vi "rasp11.vi"(7 "data type":waveform(i16)) -> (1 "element":i16)   [LabVIEW 2010]
panel:
  out "output cluster":cluster{i16[], i32[]}
  out "index":i32
  out "Waveform Graph":waveform(i16)[](graph)
  out "XY Graph":cluster{i16[], i32[]}(graph)
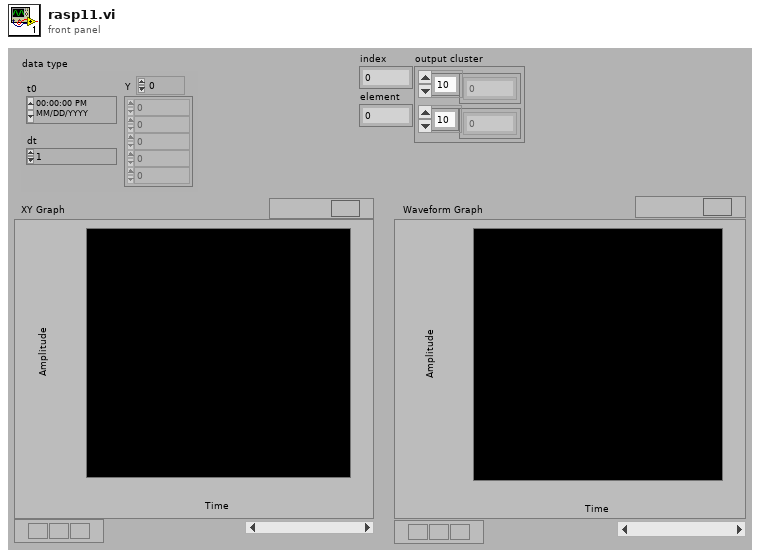
[diagram p1: front panel]
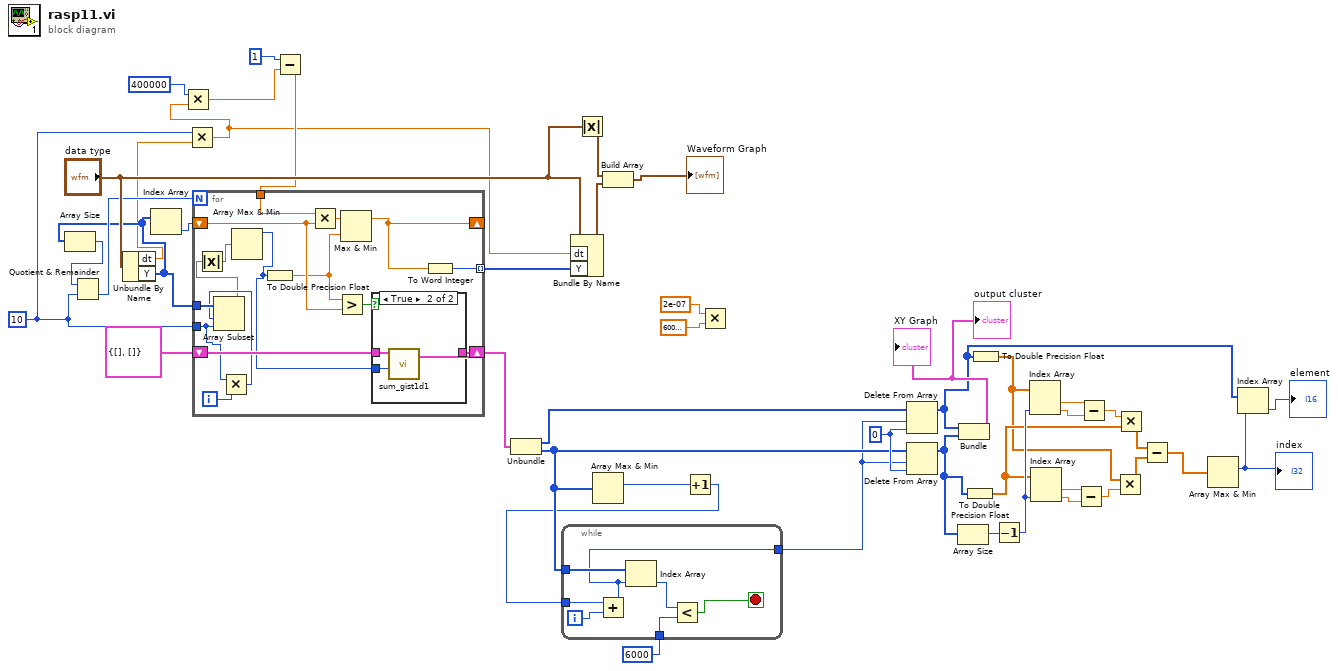
[diagram p0: block diagram]
diagram:
  w23 = 10 ("y")
  w42 = 0 ("index")
  n1 = Unbundle By Name("data type") -> ("dt"=w26:dbl, "Y"=w27:i16[])
  n2 = Array Size(array=w27) -> (size(s)=w29:i32)
  n3 = Quotient & Remainder(x=w29, y=w23) -> (floor(x/y)=w28:i32)  [unwired: 1 out]
  n4 = Index Array(array=w27) -> (element=w38:i16)  [unwired: 1 in]
  n5 = Multiply(x=w23, y=w26) -> (x*y=w1:dbl)
  n6 = Multiply(x=400000, y=w1) -> (x*y=w21:dbl)
  n7 = Subtract(x=1, y=w21) -> (x-y=w24:dbl)
  n8 = for {
    N: w28 -> [_]
    shift-right: [w54] -> _
    shift-left: w38 -> [w56]
    tunnel: [w61] -> w45 mode=indexing
    shift-right: [w59] -> w37
    shift-left: cluster{i16[], i32[]} {[], []} ("hist") -> [w60]
    tunnel: w24 -> [w53]
    tunnel: w27 -> [w52]
    tunnel: w23 -> [w50]
    i -> [w51]
    n9 = Multiply(x=w50, y=w51) -> (x*y=w49:i32)
    n10 = Array Subset(array=w52, index=w49, length=w50) -> (w48:i16[])
    n11 = Absolute Value(x=w48) -> (abs(x)=w47:i16[])
    n12 = Array Max & Min(array=w47) -> (max value=w46:i16)  [unwired: 3 out]
    n13 = To Double Precision Float(number=w46) -> (double precision float=w55:dbl)
    n14 = Multiply(x=w53, y=w56) -> (x*y=w58:dbl)
    n15 = Greater?(x=w55, y=w56) -> (0:w57:bool)
    n16 = Max & Min(x=w58, y=w55) -> (max(x,y)=w54:dbl)  [unwired: 1 out]
    n17 = case shown="True" w57 {
      tunnel: w60 -> [w62 w64]
      tunnel: w46 -> [_ w63]
      tunnel: [w62 w65] -> w59
      frame False {
      }
      frame True {
        n18 = call "sum_gist1d1.vi"("Y"=w63, "hist in"=w64) -> ("hist"=w65:cluster{i16[], i32[]})  [unwired: 3 in]
      }
    }
    n19 = To Word Integer(number=w54) -> (16bit integer=w61:i16)
  }
  n20 = Unbundle(w37) -> (w43:i16[], w36:i32[])
  n21 = Bundle By Name(cluster="data type", "dt"=w1, "Y"=w45) -> (w41:waveform(i16))
  n22 = Absolute Value(x="data type") -> (abs(x)=w40:waveform(i16))
  n23 = Array Max & Min(array=w36) -> (max index (indices)=w35:i32)  [unwired: 3 out]
  n24 = Build Array(w40, w41) -> (→"Waveform Graph":waveform(i16)[])
  n25 = Increment(x=w35) -> (x+1=w34:i32)
  n26 = while {
    tunnel: w36 -> [w72]
    tunnel: [w66] -> w33
    tunnel: 6000 ("y") -> [w70]
    tunnel: w34 -> [w67]
    i -> [w68]
    stop <- w69 stop-if-true
    n27 = Add(x=w67, y=w68) -> (x+y=w66:i32)
    n28 = Index Array(array=w72, index=w66) -> (element=w71:i32)
    n29 = Less?(x=w71, y=w70) -> (x < y?=w69:bool)
  }
  n30 = Multiply(x=2e-07, y=60000000.0) -> ()  [unwired: 1 out]
  n31 = Delete From Array(array=w43, length=w33, index=w42) -> (array with subset deleted=w5:i16[])  [unwired: 1 out]
  n32 = Delete From Array(array=w36, length=w33, index=w42) -> (array with subset deleted=w10:i32[])  [unwired: 1 out]
  n33 = Array Size(array=w10) -> (size(s)=w20:i32)
  n34 = Bundle(w5, w10) -> (→"XY Graph" →"output cluster":cluster{i16[], i32[]})  [unwired: 1 in]
  n35 = To Double Precision Float(number=w10) -> (double precision float=w9:dbl[])
  n36 = To Double Precision Float(number=w5) -> (double precision float=w8:dbl[])
  n37 = Decrement(x=w20) -> (x-1=w19:i32)
  n38 = Index Array(array=w8, index #2=w19) -> (element #1=w18:dbl, element #2=w17:dbl)  [unwired: 1 in]
  n39 = Index Array(array=w9, index #2=w19) -> (element #1=w16:dbl, element #2=w15:dbl)  [unwired: 1 in]
  n40 = Subtract(x=w16, y=w15) -> (x-y=w13:dbl)
  n41 = Subtract(x=w18, y=w17) -> (x-y=w14:dbl)
  n42 = Multiply(x=w8, y=w13) -> (x*y=w11:dbl[])
  n43 = Multiply(x=w14, y=w9) -> (x*y=w12:dbl[])
  n44 = Subtract(x=w12, y=w11) -> (x-y=w7:dbl[])
  n45 = Array Max & Min(array=w7) -> (max index (indices)=w4:i32)  [unwired: 3 out]
  "index" <- w4
  n46 = Index Array(array=w5, index=w4) -> (element=→"element":i16)
